vi "InitIO.vi"(11 "Path":path=path "IOconfig.ini") -> ()   [LabVIEW 2012]
uses:
  <vilib>/Rock Robotics/SystemInterfaces/Typedef/FPGA_TypedefDigitalModule.ctl
  <vilib>/Utility/config.llb/Read Key (Boolean).vi
  <vilib>/Utility/config.llb/Read Key (I32).vi
  <vilib>/Rock Robotics/WPI/RobotDrive/WPI_RobotDriveOpen2MotorWithVictor.vi
  <vilib>/Rock Robotics/WPI/MotorControl/WPI_MotorControlOpen Jaguar.vi
  <vilib>/Rock Robotics/WPI/Counter/WPI_CounterDigitalInputToDigitalSource.vi
  <vilib>/Rock Robotics/WPI/Counter/WPI_CounterOpen Semi Period Mode.vi
  <vilib>/Utility/config.llb/NI_LVConfig.lvlib
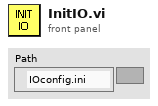
[diagram p1: front panel]
types:
  T1 = typedef "NI_LVConfig.lvlib/Config Data RefNum.ctl" = refnum<k1>
  T2 = typedef "FPGA_TypedefDigitalModule.ctl" = enum16{"Digital Module 1", "Digital Module 2"}
  T3 = typedef "WPI_MotorControlDeviceRef.ctl" = cluster{"DeviceStatus":errorcluster, "Type":enum16{"PWM", "CAN"}, "PWM":cluster{"Digital Module":T2, "PWM Channel":T4, "DeadBand":T5}, "CAN":cluster{"Device Number":u8, "Control Mode":T6, "Semaphore":T7, "Max Vout":dbl}, "Invert":bool, "TransformRef":T8, "InvTransformRef":T8}
  T4 = typedef "FPGA_DIOPWMChannel.ctl" = enum8{"PWM 1", "PWM 2", "PWM 3", "PWM 4", "PWM 5", "PWM 6", "PWM 7", "PWM 8", "PWM 9", "PWM 10", "Invalid"}
  T5 = typedef "WPI_PWMDeadband.ctl" = cluster{"Name":string, "maxPositivePwm":i32, "minPositivePwm":i32, "centerPwm":i32, "maxNegativePwm":i32, "minNegativePwm":i32, "angularRange":u16}
  T6 = typedef "WPI_CANJaguar_ControlMode.ctl" = enum8{"Percent VBus", "Current", "Speed", "Position", "Voltage"}
  T7 = typedef "Semaphore RefNum" = refnum<k1>
  T8 = typedef "WPI_PWMTransform_ConPane.ctl" = refnum<vi>
  T9 = typedef "WPI_RobotDriveDevRef.ctl" = cluster{"DevStatus":errorcluster, "Motors[]":T3[], "Square Inputs":bool, "Max Output":dbl, "Isochronous":bool}
  T10 = typedef "WPI_DigitalInputDevRef.ctl" = cluster{"DevStatus":errorcluster, "DIO Channel":T11, "Digital Module":T2}
  T11 = typedef "FPGA_DIOChannel.ctl" = enum8{"DIO 1", "DIO 2", "DIO 3", "DIO 4", "DIO 5", "DIO 6", "DIO 7", "DIO 8", "DIO 9", "DIO 10", "DIO 11", "DIO 12", "DIO 13", "DIO 14", "Invalid"}
  T12 = typedef "WPI_DigitalOutputDevRef.ctl" = cluster{"Digital Module":T2, "DIO Channel":T11, "DevStatus":errorcluster}
  T13 = typedef "FPGA_CounterEncoderSourceConvertionLVSourceType.ctl" = cluster{"DevStatus":errorcluster, "AnalogTriggerMode?":bool, "DigitalMode":cluster{"Digital Module":T2, "DIO Channel":T14}, "AnalogTriggerMode":cluster{"AnalogTriggerIndex":T15, "OutputType":T16}}
  T14 = typedef "FPGA_DIODigitalSourceChannel.ctl" = enum8{"DIO 1", "DIO 2", "DIO 3", "DIO 4", "DIO 5", "DIO 6", "DIO 7", "DIO 8", "DIO 9", "DIO 10", "DIO 11", "DIO 12", "DIO 13", "DIO 14", "Disabled"}
  T15 = typedef "FPGA_AnalogTriggerIndex.ctl" = enum8{"Trig 0", "Trig 1", "Trig 2", "Trig 3", "Trig 4", "Trig 5", "Trig 6", "Trig 7", "Invalid"}
  T16 = typedef "FPGA_AnalogTriggerOutType.ctl" = enum16{"InWindow", "TriggerState", "Rising", "Falling"}
  T17 = typedef "WPI_UltrasonicDeviceRef.ctl" = cluster{"DevStatus":errorcluster, "Ping Digital Module":T2, "Echo Digital Module":T2, "Ping Channel":T11, "Echo Channel":T11, "CntIndex":T18}
  T18 = typedef "FPGA_CounterCtrSystemIndex.ctl" = enum8{"Ctr 0", "Ctr 1", "Ctr 2", "Ctr 3", "Ctr 4", "Ctr 5", "Ctr 6", "Ctr 7", "Invalid"}
  T19 = typedef "WPI_CounterDevRef.ctl" = cluster{"DevStatus":errorcluster, "CntIndex":T18}
  T20 = typedef "WPI_EncoderDevRef.ctl" = cluster{"DevStatus":errorcluster, "EncoderIndex":T21, "CounterIndex":T18, "DistancePerCount":dbl, "Decoding Type":T22}
  T21 = typedef "FPGA_EncoderIdx.ctl" = enum8{"Enc 0", "Enc 1", "Enc 2", "Enc 3", "Invalid"}
  T22 = typedef "WPI_EncoderType.ctl" = enum16{"1x", "2x", "4x"}
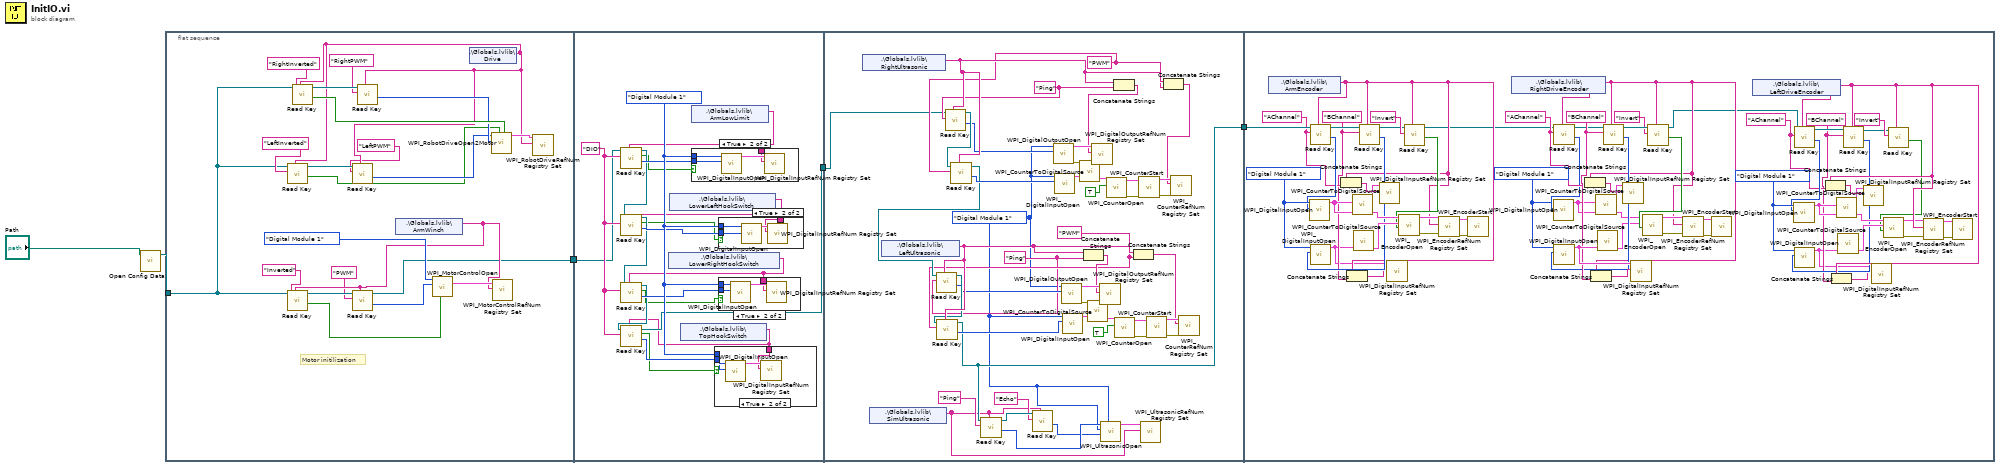
[diagram p0: block diagram]
diagram:
  n1 = call <vilib>:"Open Config Data.vi"("configuration file path"="Path") -> ("refnum"=w4:T1)  [unwired: 8 in, 2 out]
  n2 = flat-sequence {
    tunnel: w4 -> [w6]
    tunnel: [w8] -> w3
    tunnel: w3 -> [w39]
    tunnel: [w33] -> w2
    tunnel: w2 -> [w81]
    tunnel: [w71] -> w1
    tunnel: w1 -> [w160]
    frame #0 {
      # "Motor initilization"
      n3 = shared-variable ".\\Globals.lvlib\\ArmWinch"() -> (w12:string)  [unwired: 1 in, 1 out]
      n4 = call-poly <vilib>:"Read Key.vi"("section"=w12, "key"="Inverted", "refnum"=w6) -> ("value"=w10:bool, "refnum out"=w14:T1)  [unwired: 5 in, 2 out]
      n5 = call-poly <vilib>:"Read Key.vi"("section"=w12, "key"="PWM", "refnum"=w14) -> ("value"=w9:i32, "refnum out"=w8:T1)  [unwired: 5 in, 2 out]
      n6 = call-poly <vilib>:"WPI_MotorControlOpen.vi"("Invert"=w10, "PWM Channel"=w9, "Digital Module (Module 1)"=FPGA_TypedefDigitalModule."Digital Module 1") -> ("MotorControlDeviceRef"=w26:T3)  [unwired: 7 in, 1 out]
      n7 = shared-variable ".\\Globals.lvlib\\Drive"() -> (w17:string)  [unwired: 1 in, 1 out]
      n8 = call-poly <vilib>:"Read Key.vi"("section"=w17, "key"="LeftInverted", "refnum"=w6) -> ("value"=w15:bool, "refnum out"=w18:T1)  [unwired: 5 in, 2 out]
      n9 = call-poly <vilib>:"Read Key.vi"("section"=w17, "key"="RightInverted", "refnum"=w6) -> ("value"=w21:bool, "refnum out"=w24:T1)  [unwired: 5 in, 2 out]
      n10 = call-poly <vilib>:"Read Key.vi"("section"=w17, "key"="LeftPWM", "refnum"=w18) -> ("value"=w16:i32)  [unwired: 5 in, 3 out]
      n11 = call-poly <vilib>:"Read Key.vi"("section"=w17, "key"="RightPWM", "refnum"=w24) -> ("value"=w20:i32)  [unwired: 5 in, 3 out]
      n12 = call-poly <vilib>:"WPI_RobotDriveOpen2Motor.vi"("Right Motor Inverted"=w21, "Left Motor Inverted"=w15, "Right Motor"=w20, "Left Motor"=w16) -> ("RobotDriveDevRef"=w27:T9)  [unwired: 6 in, 1 out]
      n13 = call <vilib>:"WPI_MotorControlRefNum Registry Set.vi"("refnum name"=w12, "MotorControlDevRef"=w26) -> ()  [unwired: 8 in, 2 out]
      n14 = call <vilib>:"WPI_RobotDriveRefNum Registry Set.vi"("refnum name"=w17, "RobotDriveDevRef"=w27) -> ()  [unwired: 8 in, 2 out]
    }
    frame #1 {
      w40 = "DIO"
      w46 = FPGA_TypedefDigitalModule."Digital Module 1" ("Digital Module (Module 1)")
      n15 = shared-variable ".\\Globals.lvlib\\LowerRightHookSwitch"() -> (w34:string)  [unwired: 1 in, 1 out]
      n16 = shared-variable ".\\Globals.lvlib\\LowerLeftHookSwitch"() -> (w35:string)  [unwired: 1 in, 1 out]
      n17 = shared-variable ".\\Globals.lvlib\\TopHookSwitch"() -> (w32:string)  [unwired: 1 in, 1 out]
      n18 = shared-variable ".\\Globals.lvlib\\ArmLowLimit"() -> (w45:string)  [unwired: 1 in, 1 out]
      n19 = call-poly <vilib>:"Read Key.vi"("section"=w45, "key"=w40, "refnum"=w39) -> ("value"=w44:i32, "found?"=w30:bool, "refnum out"=w38:T1)  [unwired: 5 in, 1 out]
      n20 = call-poly <vilib>:"Read Key.vi"("section"=w35, "key"=w40, "refnum"=w38) -> ("value"=w41:i32, "found?"=w31:bool, "refnum out"=w37:T1)  [unwired: 5 in, 1 out]
      n21 = call-poly <vilib>:"Read Key.vi"("section"=w34, "key"=w40, "refnum"=w37) -> ("value"=w42:i32, "found?"=w29:bool, "refnum out"=w36:T1)  [unwired: 5 in, 1 out]
      n22 = call-poly <vilib>:"Read Key.vi"("section"=w32, "key"=w40, "refnum"=w36) -> ("value"=w43:i32, "found?"=w28:bool, "refnum out"=w33:T1)  [unwired: 5 in, 1 out]
      n23 = case shown="True" w30 {
        tunnel: w46 -> [_ w61]
        tunnel: w45 -> [_ w60]
        tunnel: w44 -> [_ w59]
        frame False {
        }
        frame True {
          n24 = call <vilib>:"WPI_DigitalInputOpen.vi"("DIO Channel"=w59, "Digital Module (Module 1)"=w61) -> ("DigitalInputDevRef"=w62:T10)  [unwired: 8 in, 1 out]
          n25 = call <vilib>:"WPI_DigitalInputRefNum Registry Set.vi"("refnum name"=w60, "DigitalInputDevRef"=w62) -> ()  [unwired: 8 in, 2 out]
        }
      }
      n26 = case shown="True" w28 {
        tunnel: w46 -> [_ w49]
        tunnel: w43 -> [_ w48]
        tunnel: w32 -> [_ w47]
        frame False {
        }
        frame True {
          n27 = call <vilib>:"WPI_DigitalInputOpen.vi"("DIO Channel"=w48, "Digital Module (Module 1)"=w49) -> ("DigitalInputDevRef"=w50:T10)  [unwired: 8 in, 1 out]
          n28 = call <vilib>:"WPI_DigitalInputRefNum Registry Set.vi"("refnum name"=w47, "DigitalInputDevRef"=w50) -> ()  [unwired: 8 in, 2 out]
        }
      }
      n29 = case shown="True" w31 {
        tunnel: w46 -> [_ w57]
        tunnel: w41 -> [_ w56]
        tunnel: w35 -> [_ w55]
        frame False {
        }
        frame True {
          n30 = call <vilib>:"WPI_DigitalInputOpen.vi"("DIO Channel"=w56, "Digital Module (Module 1)"=w57) -> ("DigitalInputDevRef"=w58:T10)  [unwired: 8 in, 1 out]
          n31 = call <vilib>:"WPI_DigitalInputRefNum Registry Set.vi"("refnum name"=w55, "DigitalInputDevRef"=w58) -> ()  [unwired: 8 in, 2 out]
        }
      }
      n32 = case shown="True" w29 {
        tunnel: w46 -> [_ w53]
        tunnel: w42 -> [_ w52]
        tunnel: w34 -> [_ w51]
        frame False {
        }
        frame True {
          n33 = call <vilib>:"WPI_DigitalInputOpen.vi"("DIO Channel"=w52, "Digital Module (Module 1)"=w53) -> ("DigitalInputDevRef"=w54:T10)  [unwired: 8 in, 1 out]
          n34 = call <vilib>:"WPI_DigitalInputRefNum Registry Set.vi"("refnum name"=w51, "DigitalInputDevRef"=w54) -> ()  [unwired: 8 in, 2 out]
        }
      }
    }
    frame #2 {
      w73 = "PWM"
      w72 = "Ping"
      w82 = "PWM"
      w85 = "Ping"
      w65 = FPGA_TypedefDigitalModule."Digital Module 1" ("Digital Module (Module 1)")
      n35 = shared-variable ".\\Globals.lvlib\\RightUltrasonic"() -> (w87:string)  [unwired: 1 in, 1 out]
      n36 = shared-variable ".\\Globals.lvlib\\SimUltrasonic"() -> (w63:string)  [unwired: 1 in, 1 out]
      n37 = shared-variable ".\\Globals.lvlib\\LeftUltrasonic"() -> (w78:string)  [unwired: 1 in, 1 out]
      n38 = call-poly <vilib>:"Read Key.vi"("section"=w87, "key"=w85, "refnum"=w81) -> ("value"=w84:i32, "refnum out"=w86:T1)  [unwired: 5 in, 2 out]
      n39 = call-poly <vilib>:"Read Key.vi"("section"=w87, "key"=w82, "refnum"=w86) -> ("value"=w83:i32, "refnum out"=w77:T1)  [unwired: 5 in, 2 out]
      n40 = call-poly <vilib>:"Read Key.vi"("section"=w78, "key"=w72, "refnum"=w77) -> ("value"=w74:i32, "refnum out"=w76:T1)  [unwired: 5 in, 2 out]
      n41 = call-poly <vilib>:"Read Key.vi"("section"=w78, "key"=w73, "refnum"=w76) -> ("value"=w75:i32, "refnum out"=w71:T1)  [unwired: 5 in, 2 out]
      n42 = call-poly <vilib>:"Read Key.vi"("section"=w63, "key"="Ping", "refnum"=w71) -> ("value"=w68:i32, "refnum out"=w70:T1)  [unwired: 5 in, 2 out]
      n43 = call-poly <vilib>:"Read Key.vi"("section"=w63, "key"="Echo", "refnum"=w70) -> ("value"=w67:i32)  [unwired: 5 in, 3 out]
      n44 = call <vilib>:"WPI_DigitalOutputOpen.vi"("DIO Channel"=w84, "Digital Module (Module 1)"=w65) -> ("error out"=w98:errorcluster, "DigitalOutputDevRef"=w97:T12)  [unwired: 8 in]
      n45 = call <vilib>:"WPI_DigitalInputOpen.vi"("DIO Channel"=w83, "Digital Module (Module 1)"=w65) -> ("DigitalInputDevRef"=w96:T10)  [unwired: 8 in, 1 out]
      n46 = call <vilib>:"WPI_DigitalOutputOpen.vi"("DIO Channel"=w74, "Digital Module (Module 1)"=w65) -> ("error out"=w99:errorcluster, "DigitalOutputDevRef"=w100:T12)  [unwired: 8 in]
      n47 = call <vilib>:"WPI_DigitalInputOpen.vi"("DIO Channel"=w75, "Digital Module (Module 1)"=w65) -> ("DigitalInputDevRef"=w101:T10)  [unwired: 8 in, 1 out]
      n48 = call-poly <vilib>:"WPI_CounterToDigitalSource.vi"("DigitalInputDevRef"=w96) -> ("Digital Source"=w95:T13)  [unwired: 6 in]
      n49 = Concatenate Strings(w78, w72) -> (w80:string)
      n50 = call-poly <vilib>:"WPI_CounterToDigitalSource.vi"("DigitalInputDevRef"=w101) -> ("Digital Source"=w102:T13)  [unwired: 6 in]
      n51 = call <vilib>:"WPI_DigitalOutputRefNum Registry Set.vi"("error in (no error)"=w99, "refnum name"=w80, "DigitalOutputDevRef"=w100) -> ()  [unwired: 7 in, 2 out]
      n52 = call <vilib>:"WPI_UltrasonicOpen.vi"("Ping Digital Module (Module 1)"=w65, "Echo DIO Channel"=w67, "Echo Digital Module (Module 1)"=w65, "Ping DIO Channel"=w68) -> ("UltrasonicDevRef"=w64:T17)  [unwired: 6 in, 1 out]
      n53 = call-poly <vilib>:"WPI_CounterOpen.vi"("High Pulse (T)"=TRUE, "Source"=w95) -> ("error out"=w93:errorcluster, "CounterDevRef"=w92:T19)  [unwired: 8 in]
      n54 = Concatenate Strings(w87, w85) -> (w89:string)
      n55 = call <vilib>:"WPI_DigitalOutputRefNum Registry Set.vi"("error in (no error)"=w98, "refnum name"=w89, "DigitalOutputDevRef"=w97) -> ()  [unwired: 7 in, 2 out]
      n56 = call-poly <vilib>:"WPI_CounterOpen.vi"("High Pulse (T)"=TRUE, "Source"=w102) -> ("error out"=w104:errorcluster, "CounterDevRef"=w105:T19)  [unwired: 8 in]
      n57 = Concatenate Strings(w78, w73) -> (w79:string)
      n58 = call <vilib>:"WPI_CounterStart.vi"("error in (no error)"=w93, "CounterDevRef in"=w92) -> ("error out"=w91:errorcluster, "CounterDevRef out"=w90:T19)  [unwired: 8 in]
      n59 = call <vilib>:"WPI_UltrasonicRefNum Registry Set.vi"("refnum name"=w63, "UltrasonicDevRef"=w64) -> ()  [unwired: 8 in, 2 out]
      n60 = call <vilib>:"WPI_CounterStart.vi"("error in (no error)"=w104, "CounterDevRef in"=w105) -> ("error out"=w106:errorcluster, "CounterDevRef out"=w107:T19)  [unwired: 8 in]
      n61 = Concatenate Strings(w87, w82) -> (w88:string)
      n62 = call <vilib>:"WPI_CounterRefNum Registry Set.vi"("error in (no error)"=w91, "refnum name"=w88, "CounterDevRef"=w90) -> ()  [unwired: 7 in, 2 out]
      n63 = call <vilib>:"WPI_CounterRefNum Registry Set.vi"("error in (no error)"=w106, "refnum name"=w79, "CounterDevRef"=w107) -> ()  [unwired: 7 in, 2 out]
    }
    frame #3 {
      w110 = "BChannel"
      w112 = "AChannel"
      w127 = FPGA_TypedefDigitalModule."Digital Module 1" ("Digital Module (Module 1)")
      w148 = "BChannel"
      w146 = "AChannel"
      w131 = FPGA_TypedefDigitalModule."Digital Module 1" ("Digital Module (Module 1)")
      w151 = "BChannel"
      w154 = "AChannel"
      w170 = FPGA_TypedefDigitalModule."Digital Module 1" ("Digital Module (Module 1)")
      n64 = shared-variable ".\\Globals.lvlib\\ArmEncoder"() -> (w152:string)  [unwired: 1 in, 1 out]
      n65 = call-poly <vilib>:"Read Key.vi"("section"=w152, "key"=w154, "refnum"=w160) -> ("value"=w159:i32, "refnum out"=w161:T1)  [unwired: 5 in, 2 out]
      n66 = call <vilib>:"WPI_DigitalInputOpen.vi"("DIO Channel"=w159, "Digital Module (Module 1)"=w170) -> ("DigitalInputDevRef"=w155:T10)  [unwired: 8 in, 1 out]
      n67 = Concatenate Strings(w152, w154) -> (w156:string)
      n68 = Concatenate Strings(w152, w151) -> (w153:string)
      n69 = call-poly <vilib>:"WPI_CounterToDigitalSource.vi"("DigitalInputDevRef"=w155) -> ("Digital Source"=w166:T13)  [unwired: 6 in]
      n70 = call-poly <vilib>:"Read Key.vi"("section"=w152, "key"=w151, "refnum"=w161) -> ("value"=w158:i32, "refnum out"=w162:T1)  [unwired: 5 in, 2 out]
      n71 = call <vilib>:"WPI_DigitalInputOpen.vi"("DIO Channel"=w158, "Digital Module (Module 1)"=w170) -> ("DigitalInputDevRef"=w150:T10)  [unwired: 8 in, 1 out]
      n72 = call-poly <vilib>:"WPI_CounterToDigitalSource.vi"("DigitalInputDevRef"=w150) -> ("Digital Source"=w167:T13)  [unwired: 6 in]
      n73 = call <vilib>:"WPI_DigitalInputRefNum Registry Set.vi"("refnum name"=w156, "DigitalInputDevRef"=w155) -> ()  [unwired: 8 in, 2 out]
      n74 = call <vilib>:"WPI_DigitalInputRefNum Registry Set.vi"("refnum name"=w153, "DigitalInputDevRef"=w150) -> ()  [unwired: 8 in, 2 out]
      n75 = call-poly <vilib>:"Read Key.vi"("section"=w152, "key"="Invert", "refnum"=w162) -> ("value"=w157:bool, "refnum out"=w130:T1)  [unwired: 5 in, 2 out]
      n76 = call <vilib>:"WPI_EncoderOpen.vi"("Invert Direction (False)"=w157, "BSource"=w167, "ASource"=w166) -> ("error out"=w165:errorcluster, "EncoderDevRef"=w168:T20)  [unwired: 7 in]
      n77 = call <vilib>:"WPI_EncoderRefNum Registry Set.vi"("error in (no error)"=w165, "refnum name"=w152, "EncoderDevRef"=w168) -> ("error out"=w164:errorcluster, "EncoderDevRef"=w169:T20)  [unwired: 7 in]
      n78 = call <vilib>:"WPI_EncoderStart.vi"("error in (no error)"=w164, "EncoderDevRef"=w169) -> ()  [unwired: 8 in, 2 out]
      n79 = shared-variable ".\\Globals.lvlib\\RightDriveEncoder"() -> (w129:string)  [unwired: 1 in, 1 out]
      n80 = call-poly <vilib>:"Read Key.vi"("section"=w129, "key"=w146, "refnum"=w130) -> ("value"=w141:i32, "refnum out"=w140:T1)  [unwired: 5 in, 2 out]
      n81 = call <vilib>:"WPI_DigitalInputOpen.vi"("DIO Channel"=w141, "Digital Module (Module 1)"=w131) -> ("DigitalInputDevRef"=w145:T10)  [unwired: 8 in, 1 out]
      n82 = Concatenate Strings(w129, w146) -> (w144:string)
      n83 = Concatenate Strings(w129, w148) -> (w147:string)
      n84 = call-poly <vilib>:"WPI_CounterToDigitalSource.vi"("DigitalInputDevRef"=w145) -> ("Digital Source"=w135:T13)  [unwired: 6 in]
      n85 = call-poly <vilib>:"Read Key.vi"("section"=w129, "key"=w148, "refnum"=w140) -> ("value"=w142:i32, "refnum out"=w139:T1)  [unwired: 5 in, 2 out]
      n86 = call <vilib>:"WPI_DigitalInputOpen.vi"("DIO Channel"=w142, "Digital Module (Module 1)"=w131) -> ("DigitalInputDevRef"=w149:T10)  [unwired: 8 in, 1 out]
      n87 = call-poly <vilib>:"WPI_CounterToDigitalSource.vi"("DigitalInputDevRef"=w149) -> ("Digital Source"=w134:T13)  [unwired: 6 in]
      n88 = call <vilib>:"WPI_DigitalInputRefNum Registry Set.vi"("refnum name"=w144, "DigitalInputDevRef"=w145) -> ()  [unwired: 8 in, 2 out]
      n89 = call <vilib>:"WPI_DigitalInputRefNum Registry Set.vi"("refnum name"=w147, "DigitalInputDevRef"=w149) -> ()  [unwired: 8 in, 2 out]
      n90 = call-poly <vilib>:"Read Key.vi"("section"=w129, "key"="Invert", "refnum"=w139) -> ("value"=w143:bool, "refnum out"=w108:T1)  [unwired: 5 in, 2 out]
      n91 = call <vilib>:"WPI_EncoderOpen.vi"("Invert Direction (False)"=w143, "BSource"=w134, "ASource"=w135) -> ("error out"=w136:errorcluster, "EncoderDevRef"=w133:T20)  [unwired: 7 in]
      n92 = call <vilib>:"WPI_EncoderRefNum Registry Set.vi"("error in (no error)"=w136, "refnum name"=w129, "EncoderDevRef"=w133) -> ("error out"=w137:errorcluster, "EncoderDevRef"=w132:T20)  [unwired: 7 in]
      n93 = call <vilib>:"WPI_EncoderStart.vi"("error in (no error)"=w137, "EncoderDevRef"=w132) -> ()  [unwired: 8 in, 2 out]
      n94 = shared-variable ".\\Globals.lvlib\\LeftDriveEncoder"() -> (w128:string)  [unwired: 1 in, 1 out]
      n95 = call-poly <vilib>:"Read Key.vi"("section"=w128, "key"=w112, "refnum"=w108) -> ("value"=w117:i32, "refnum out"=w118:T1)  [unwired: 5 in, 2 out]
      n96 = call <vilib>:"WPI_DigitalInputOpen.vi"("DIO Channel"=w117, "Digital Module (Module 1)"=w127) -> ("DigitalInputDevRef"=w113:T10)  [unwired: 8 in, 1 out]
      n97 = Concatenate Strings(w128, w112) -> (w114:string)
      n98 = Concatenate Strings(w128, w110) -> (w111:string)
      n99 = call-poly <vilib>:"WPI_CounterToDigitalSource.vi"("DigitalInputDevRef"=w113) -> ("Digital Source"=w123:T13)  [unwired: 6 in]
      n100 = call-poly <vilib>:"Read Key.vi"("section"=w128, "key"=w110, "refnum"=w118) -> ("value"=w116:i32, "refnum out"=w119:T1)  [unwired: 5 in, 2 out]
      n101 = call <vilib>:"WPI_DigitalInputOpen.vi"("DIO Channel"=w116, "Digital Module (Module 1)"=w127) -> ("DigitalInputDevRef"=w109:T10)  [unwired: 8 in, 1 out]
      n102 = call-poly <vilib>:"WPI_CounterToDigitalSource.vi"("DigitalInputDevRef"=w109) -> ("Digital Source"=w124:T13)  [unwired: 6 in]
      n103 = call <vilib>:"WPI_DigitalInputRefNum Registry Set.vi"("refnum name"=w114, "DigitalInputDevRef"=w113) -> ()  [unwired: 8 in, 2 out]
      n104 = call <vilib>:"WPI_DigitalInputRefNum Registry Set.vi"("refnum name"=w111, "DigitalInputDevRef"=w109) -> ()  [unwired: 8 in, 2 out]
      n105 = call-poly <vilib>:"Read Key.vi"("section"=w128, "key"="Invert", "refnum"=w119) -> ("value"=w115:bool)  [unwired: 5 in, 3 out]
      n106 = call <vilib>:"WPI_EncoderOpen.vi"("Invert Direction (False)"=w115, "BSource"=w124, "ASource"=w123) -> ("error out"=w122:errorcluster, "EncoderDevRef"=w125:T20)  [unwired: 7 in]
      n107 = call <vilib>:"WPI_EncoderRefNum Registry Set.vi"("error in (no error)"=w122, "refnum name"=w128, "EncoderDevRef"=w125) -> ("error out"=w121:errorcluster, "EncoderDevRef"=w126:T20)  [unwired: 7 in]
      n108 = call <vilib>:"WPI_EncoderStart.vi"("error in (no error)"=w121, "EncoderDevRef"=w126) -> ()  [unwired: 8 in, 2 out]
    }
  }
